vi "CAN Monitor.vi"() -> ()   [LabVIEW 2015]
uses:
  <vilib>/Platform/TimedLoop/XDataNode/timing_clust.ctl
  <vilib>/Platform/TimedLoop/XDataNode/nitl_modes.ctl
  <vilib>/Platform/TimedLoop/XDataNode/wakeup.ctl
  <vilib>/Platform/TimedLoop/XDataNode/XDataNode.xnode
  <vilib>/Platform/TimedLoop/XDataNode/XDNodeRunTimeDep.lvlib
panel:
  out "Array":u32[](array[numeric])
  out "identifier":u32
  out "Stop Out":bool
  out "Waveform Chart":i32(graph)
  out "Messages Received":i32
  out "payload":u8[](array[numeric])
  out "Elapsed Time":dbl
  out "Messages/second":dbl
  in  "Stop":bool
  out "error out":errorcluster
  out "Messages":i32
  in  "Baud Rate":u32=1000000
  # "REALTIME"
  # "AFTER EXIT"
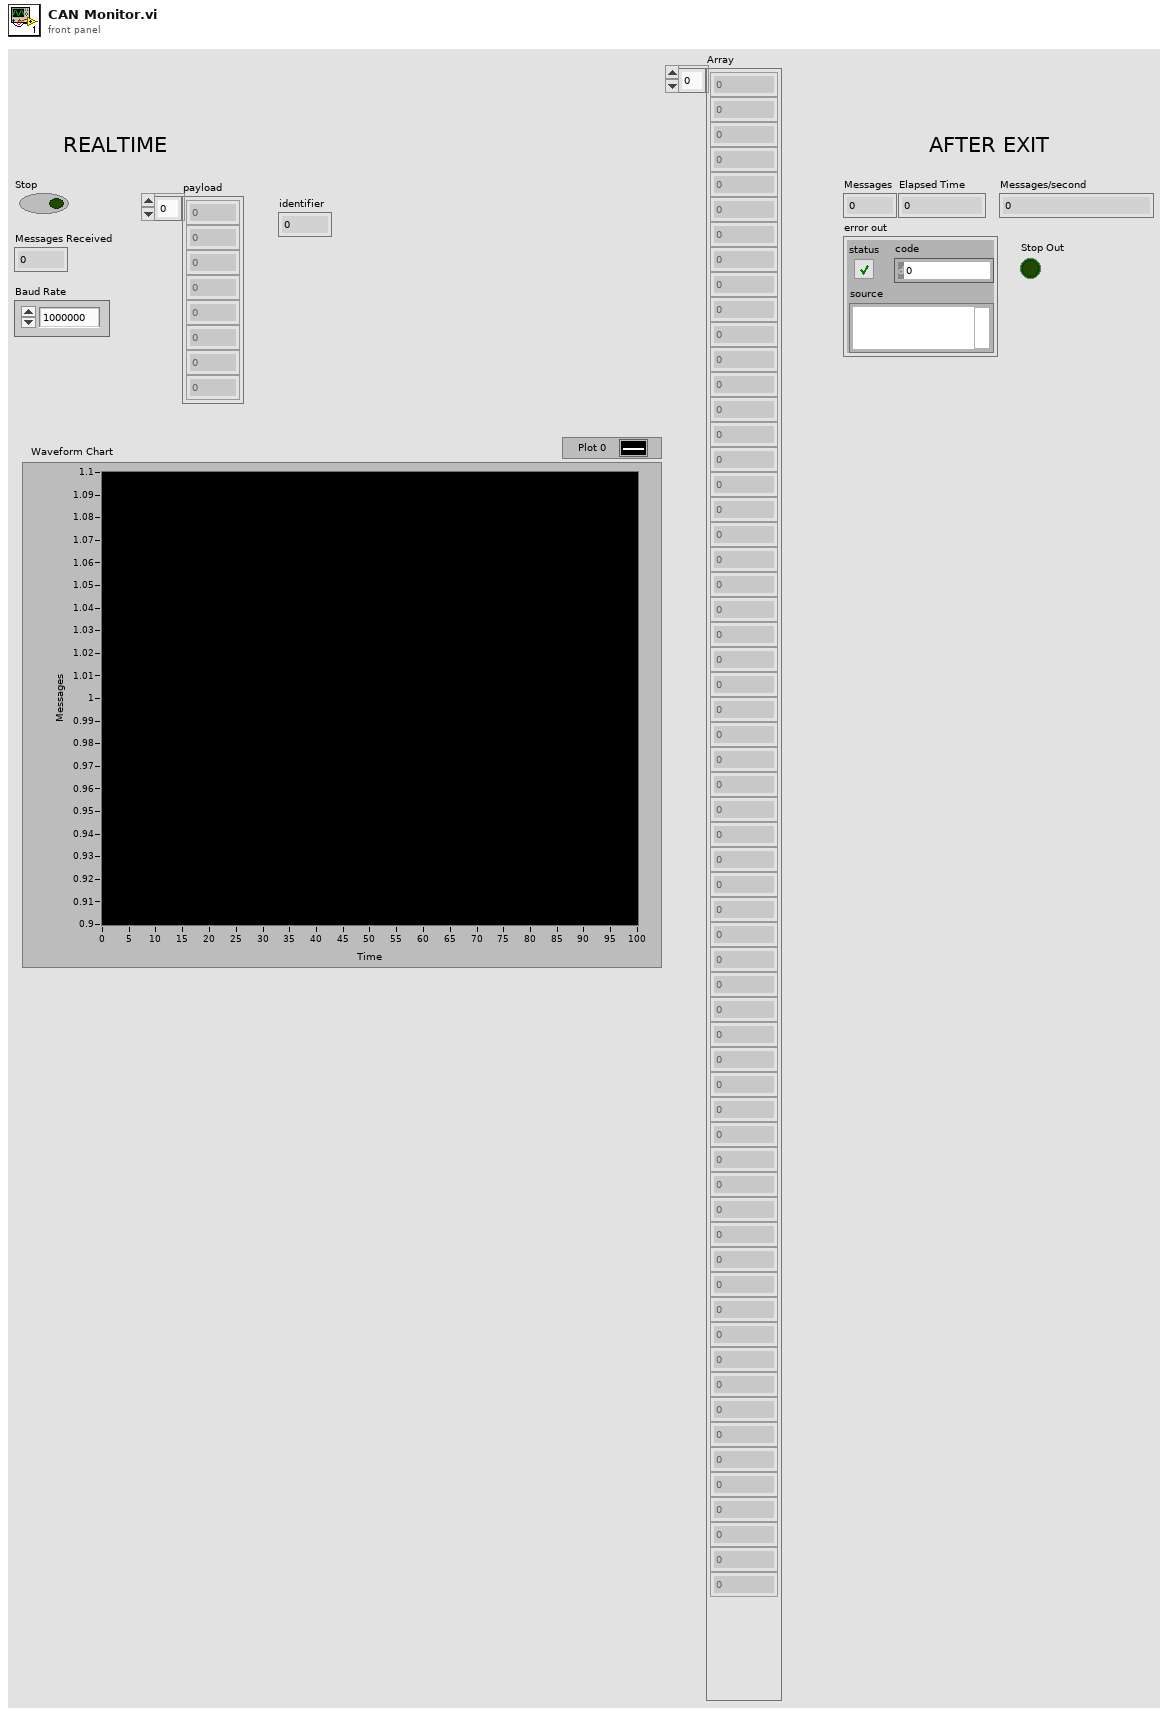
[diagram p1: front panel]
types:
  T1 = typedef "XDNodeRunTimeDep.lvlib/timing_clust.ctl" = cluster{"Expected End [f-1]":u64, "Actual End [f-1]":u64, "Finished Late? [f-1]":bool, "Expected End [i-1]":u64, "Actual End [i-1]":u64, "Finished Late? [i-1]":bool, "Expected Start [i]":u64, "Actual Start [i]":u64, "Expected Start [f]":u64, "Actual Start [f]":u64, "Source Name":string, "Structure Name":string, "Period":i64, "Deadline":i64, "Offset":i64, "Start":i64, "Priority":i32, "Timeout":i32, "Mode":T2, "Wakeup Reason":T3, "Error":errorcluster, "Source Type":string, "Secondary Source Type":string, "Global End Time":u64, "Global Start Time":u64, "Frame Duration":u64, "Iteration Duration":u64, "Assigned CPU":i32, "I/O Scan Engine Mode":u32}
  T2 = typedef "XDNodeRunTimeDep.lvlib/nitl_modes.ctl" = enum32{"No Change", "Process missed periods, maintain original phase", "Discard missed periods, maintain original phase", "Process missed periods, ignore original phase", "Discard missed periods, ignore original phase"}
  T3 = typedef "XDNodeRunTimeDep.lvlib/wakeup.ctl" = enum32{"Normal", "Aborted", "Asynchronous wakeup", "Timing source error", "Timed loop error", "Timeout"}
  T4 = typedef "CANFrameControl.ctl" = cluster{"identifier":u32, "extended?":bool, "type":u8, "payload":u8[]}
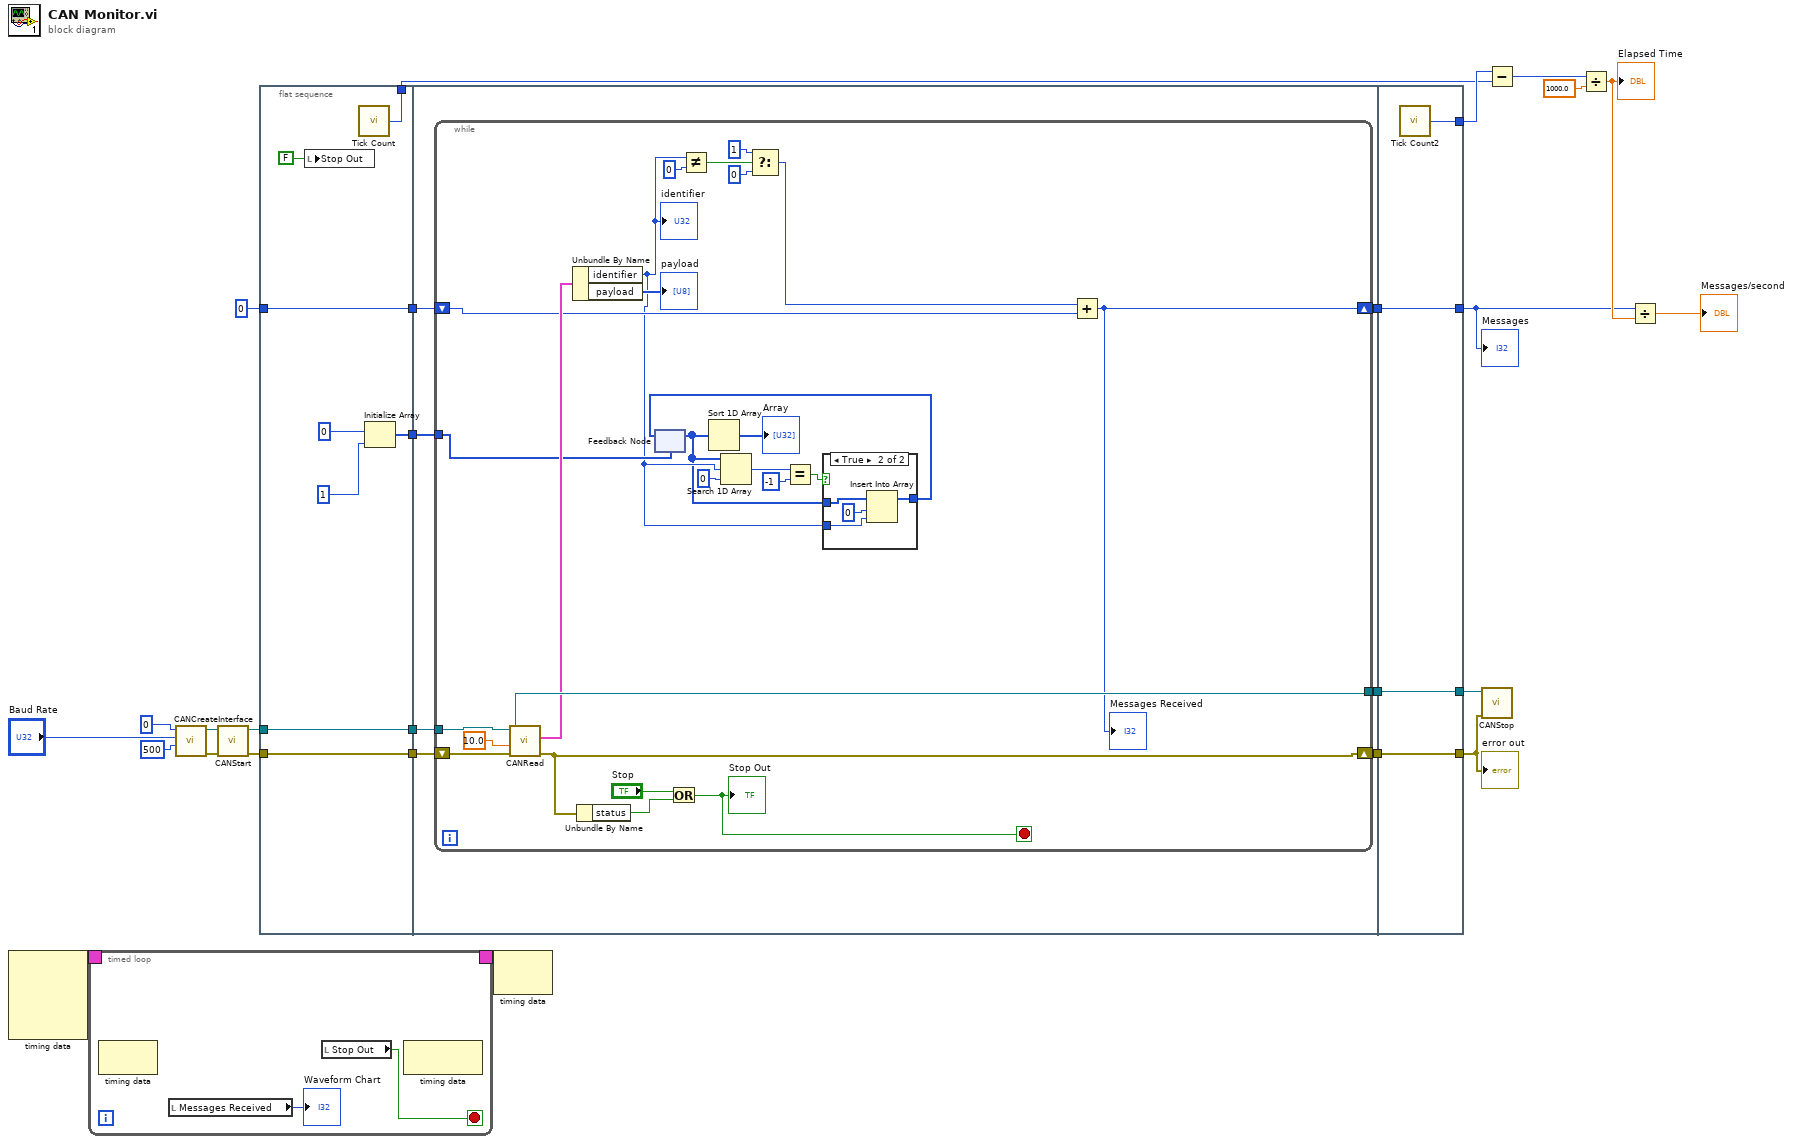
[diagram p0: block diagram]
diagram:
  n1 = node-c288() -> (w3:T1)  [unwired: 4 in]
  n2 = timed-loop {
    timing: w3 -> [_]
    timing-out: [_] -> w2
    stop <- w27 stop-if-true
    n3 = node-c288() -> ()  [unwired: 1 in, 1 out]
    n4 = local read "Messages Received"() -> (→"Waveform Chart":i32)
    n5 = local read "Stop Out"() -> (w27:bool)
    n6 = node-c288() -> ()  [unwired: 1 in, 1 out]
  }
  n7 = call <vilib>:"CANCreateInterface.vi"("receive queue size (5)"=u32 500, "baud rate (125000 bps)"="Baud Rate", "interface index"=u32 0) -> ("error out"=w26:errorcluster, "interface object out"=w25:refnum<k20>)  [unwired: 7 in]
  n8 = call <vilib>:"CANStart.vi"("error in (no error)"=w26, "interface object in"=w25) -> ("error out"=w18:errorcluster, "interface object out"=w24:refnum<k20>)  [unwired: 8 in]
  n9 = flat-sequence {
    tunnel: w18 -> [w36]
    tunnel: 0 ("index") -> [w37]
    tunnel: w24 -> [w38]
    tunnel: [w38] -> w11
    tunnel: [w37] -> w10
    tunnel: [w36] -> w9
    tunnel: [w35] -> w4
    tunnel: [w31] -> w1
    tunnel: w11 -> [w45]
    tunnel: w10 -> [w42]
    tunnel: w9 -> [w41]
    tunnel: [w44] -> w8
    tunnel: [w43] -> w7
    tunnel: [w40] -> w6
    tunnel: w1 -> [w39]
    tunnel: [w78] -> w13
    tunnel: [w79] -> w22
    tunnel: [w80] -> w23
    tunnel: w8 -> [w80]
    tunnel: w7 -> [w79]
    tunnel: w6 -> [w78]
    tunnel: [w77] -> w5
    frame #0 {
      n10 = local write "Stop Out"(FALSE ("Stop Out")) -> ()
      n11 = call "Tick Count"() -> ("Tick Count(mSec)"=w35:u32)
      n12 = Initialize Array(u32 0, 1) -> (w31:u32[])
    }
    frame #1 {
      n13 = while {
        tunnel: w45 -> [w46]
        tunnel: [w71] -> w44
        shift-right: [w57] -> w40
        shift-left: w42 -> [w61]
        shift-right: [w67] -> w43
        shift-left: w41 -> [w68]
        tunnel: w39 -> [w54]
        stop <- w56 stop-if-true
        n14 = call <vilib>:"CANRead.vi"("error in (no error)"=w68, "timeout (0 s)"=10.0, "interface object in"=w46) -> ("error out"=w67:errorcluster, "CAN frame"=w70:T4, "interface object out"=w71:refnum<k20>)  [unwired: 5 in, 1 out]
        n15 = Unbundle By Name(w70) -> ("identifier"=w53:u32, "payload"=→"payload":u8[])
        "identifier" <- w53
        n16 = Unbundle By Name(w67) -> ("status"=w66:bool)
        n17 = feedback #1(w54) -> (w48:u32[])
        n18 = Or(x="Stop", y=w66) -> (x .or. y?=w56:bool)
        "Stop Out" <- w56
        n19 = Not Equal?(x=w53, y=u32 0) -> (x != y?=w63:bool)
        n20 = Sort 1D Array(array=w48) -> (sorted array=→"Array":u32[])
        n21 = Search 1D Array(1D array=w48, element=w53, start index (0)=u32 0) -> (index of element=w52:i32)
        n22 = Select(t=1, s=w63, f=0 ("index")) -> (s? t:f=w62:i32)
        n23 = Equal?(x=w52, y=-1) -> (x = y?=w50:bool)
        n24 = case shown="True" w50 {
          tunnel: w53 -> [_ w76]
          tunnel: [w72 w75] -> w55
          tunnel: w48 -> [w72 w74]
          frame False {
          }
          frame True {
            n25 = Insert Into Array(array=w74, index=u32 0, new element=w76) -> (w75:u32[])
          }
        }
        n26 = feedback-in #1(w55) -> ()
        n27 = Add(x=w62, y=w61) -> (x+y=w57:i32)
        "Messages Received" <- w57
      }
    }
    frame #2 {
      n28 = call "Tick Count2"() -> ("Tick Count(mSec)"=w77:u32)
    }
  }
  n29 = node-c288(w2) -> ()  [unwired: 1 out]
  n30 = call <vilib>:"CANStop.vi"("error in (no error)"=w22, "interface object in"=w23) -> ()  [unwired: 8 in, 2 out]
  n31 = Subtract(x=w5, y=w4) -> (x-y=w16:u32)
  n32 = Divide(x=w16, y=1000.0) -> (x/y=w14:dbl)
  "Elapsed Time" <- w14
  n33 = Divide(x=w13, y=w14) -> (x/y=→"Messages/second":dbl)
  "Messages" <- w13
  "error out" <- w22
